vi "e_guidance (SubVI).vi"(9 "Position (i+1)":T1, 10 "Time":T2, 11 "Data":dbl[][](array[numeric])) -> (3 "e(i+1)":dbl[](array[numeric]))   [LabVIEW 2017]
uses:
  <vilib>/Analysis/_algsub.llb/Vector Norm Type.ctl
  <vilib>/Analysis/_algsub.llb/Real Vector Norm.vi
  <vilib>/Analysis/baseanly.llb/Mean (DBL).vi
  <vilib>/Analysis/baseanly.llb/Real Dot Product.vi
  <vilib>/Analysis/Matrix/Numeric/Conversions/Array To Matrix - RA2.vi
  <vilib>/Analysis/Matrix/Numeric/Conversions/Matrix To Array - RM.vi
  <vilib>/Analysis/NI_AALPro.lvlib
  <vilib>/Analysis/NI_AALBase.lvlib
  <vilib>/Analysis/Matrix/NI_Matrix.lvlib
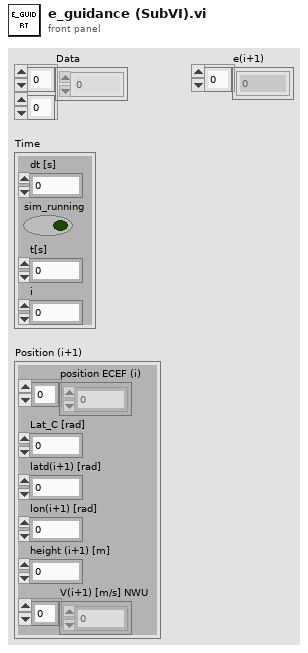
[diagram p1: front panel]
types:
  T1 = cluster{"position ECEF (i)":dbl[], "Lat_C [rad]":dbl, "latd(i+1) [rad]":dbl, "lon(i+1) [rad]":dbl, "height (i+1) [m]":dbl, "V(i+1) [m/s] NWU":dbl[]}
  T2 = cluster{"dt [s]":dbl, "sim_running":bool, "t[s]":dbl, "i":i32}
  T3 = typedef "NI_AALPro.lvlib/Vector Norm Type.ctl" = u16
  T4 = typedef "NI_Matrix.lvlib/RealMatrix.ctl" = dbl[][]
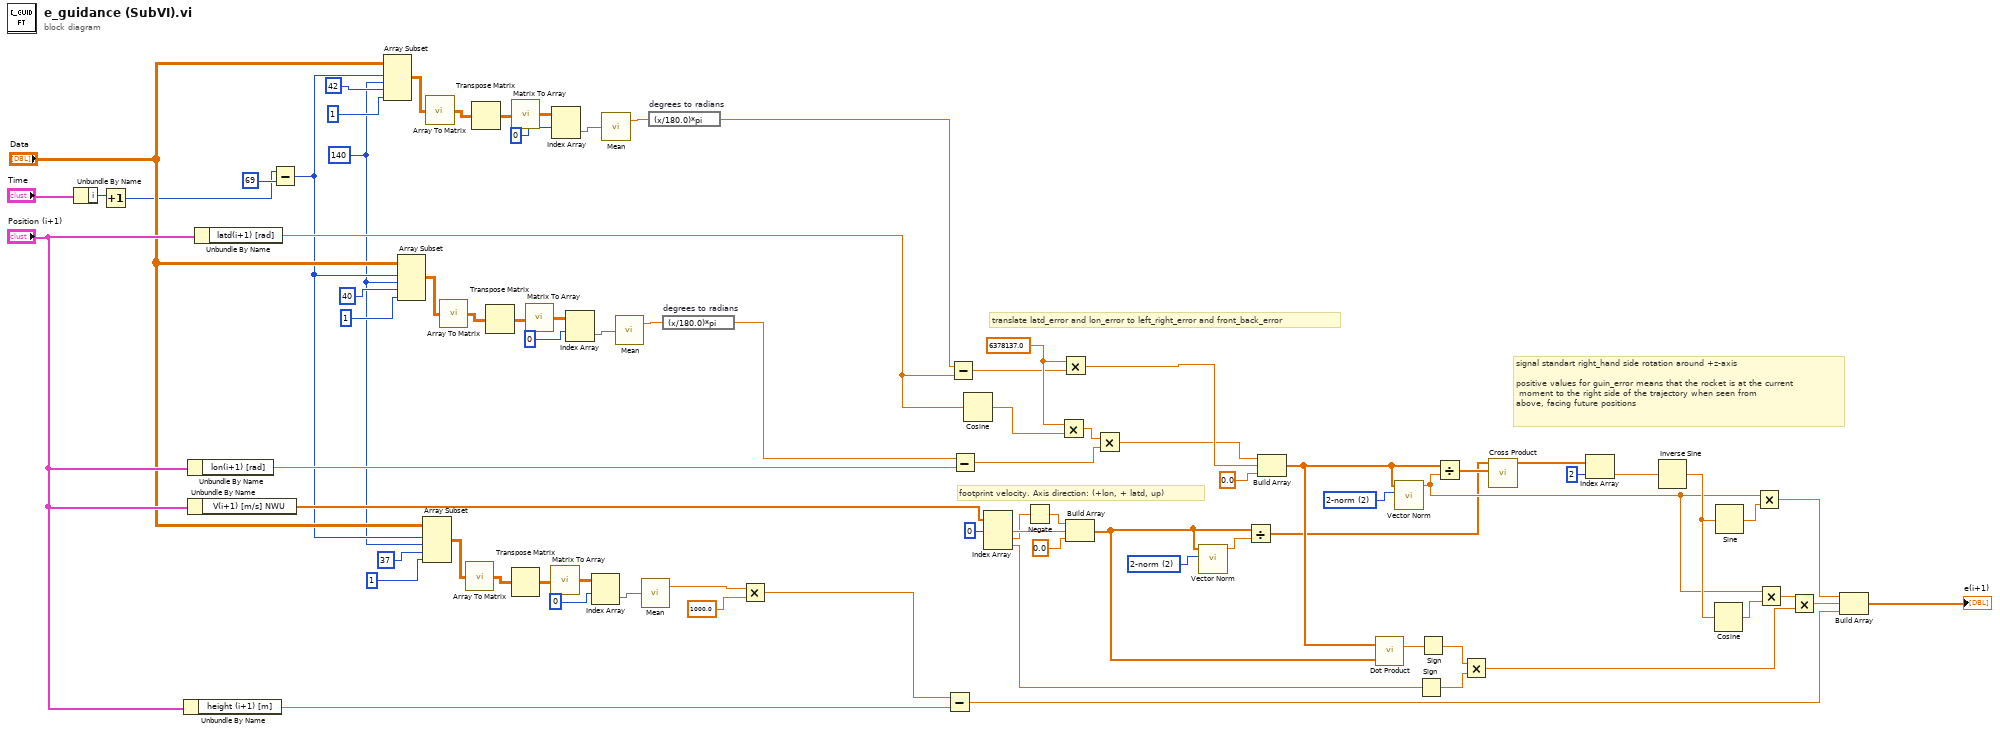
[diagram p0: block diagram]
diagram:
  w6 = 140 ("length")
  w56 = T3 2 items=["1-norm"=1, "2-norm"=2, "Inf-norm"=3, "-Inf-norm"=4, "User Defined"=5] ("norm type")
  w54 = T3 2 items=["1-norm"=1, "2-norm"=2, "Inf-norm"=3, "-Inf-norm"=4, "User Defined"=5] ("norm type")
  w41 = 6378137.0 ("x")
  # "signal standart right_hand side rotation around +z-axis\n\npositive values for guin_error means that the rocket is at the current\n moment to the right side of the trajectory when seen from \nabove, facing future positions"
  # "footprint velocity. Axis direction: (+lon, + latd, up)"
  # "translate latd_error and lon_error to left_right_error and front_back_error"
  n1 = Unbundle By Name("Time") -> ("i"=w74:i32)
  n2 = Increment(x=w74) -> (x+1=w7:i32)
  n3 = Unbundle By Name("Position (i+1)") -> ("height (i+1) [m]"=w75:dbl)
  n4 = Unbundle By Name("Position (i+1)") -> ("lon(i+1) [rad]"=w38:dbl)
  n5 = Unbundle By Name("Position (i+1)") -> ("V(i+1) [m/s] NWU"=w48:dbl[])
  n6 = Unbundle By Name("Position (i+1)") -> ("latd(i+1) [rad]"=w40:dbl)
  n7 = Subtract(x=w7, y=69) -> (x-y=w8:i32)
  n8 = Array Subset(array="Data", index (row)=w8, length (row)=w6, index (col)=42 ("index"), length (col)=1 ("length")) -> (w28:dbl[][])
  n9 = Array Subset(array="Data", index (row)=w8, length (row)=w6, index (col)=40 ("index"), length (col)=1 ("length")) -> (w24:dbl[][])
  n10 = Array Subset(array="Data", index (row)=w8, length (row)=w6, index (col)=37 ("index"), length (col)=1 ("length")) -> (w11:dbl[][])
  n11 = call-poly <vilib>:"Array To Matrix.vi"("Real 2D Array"=w28) -> ("Real Matrix"=w32:T4)
  n12 = call-poly <vilib>:"Array To Matrix.vi"("Real 2D Array"=w24) -> ("Real Matrix"=w21:T4)
  n13 = call-poly <vilib>:"Array To Matrix.vi"("Real 2D Array"=w11) -> ("Real Matrix"=w14:T4)
  n14 = Transpose Matrix(1:w32) -> (0:w31:T4)
  n15 = Transpose Matrix(1:w21) -> (0:w22:T4)
  n16 = call-poly <vilib>:"Matrix To Array.vi"("Real Matrix"=w31) -> ("Real 2D Array"=w30:dbl[][])
  n17 = Transpose Matrix(1:w14) -> (0:w13:T4)
  n18 = call-poly <vilib>:"Matrix To Array.vi"("Real Matrix"=w22) -> ("Real 2D Array"=w23:dbl[][])
  n19 = call-poly <vilib>:"Matrix To Array.vi"("Real Matrix"=w13) -> ("Real 2D Array"=w12:dbl[][])
  n20 = Index Array(array=w30, index (row)=0) -> (element=w27:dbl[])  [unwired: 1 in]
  n21 = Index Array(array=w23, index (row)=0) -> (element=w25:dbl[])  [unwired: 1 in]
  n22 = Index Array(array=w12, index (row)=0) -> (element=w10:dbl[])  [unwired: 1 in]
  n23 = call-poly <vilib>:"Mean.vi"("X"=w27) -> ("mean"=w5:dbl)  [unwired: 1 out]
  n24 = call-poly <vilib>:"Mean.vi"("X"=w25) -> ("mean"=w4:dbl)  [unwired: 1 out]
  n25 = call-poly <vilib>:"Mean.vi"("X"=w10) -> ("mean"=w2:dbl)  [unwired: 1 out]
  n26 = expression code="(x/180.0)*pi" "degrees to radians"(w5) -> (w26:dbl)
  n27 = expression code="(x/180.0)*pi" "degrees to radians"(w4) -> (w36:dbl)
  n28 = Multiply(x=w2, y=1000.0) -> (x*y=w1:dbl)
  n29 = Subtract(x=w1, y=w75) -> (x-y=w79:dbl)
  n30 = Subtract(x=w26, y=w40) -> (x-y=w39:dbl)
  n31 = Subtract(x=w36, y=w38) -> (x-y=w44:dbl)
  n32 = Cosine(x=w40) -> (cos(x)=w42:dbl)
  n33 = Index Array(array=w48, index #1=0 ("index")) -> (element #1=w52:dbl, element #2=w51:dbl, element #3=w69:dbl)  [unwired: 2 in]
  n34 = Negate(x=w51) -> (-x=w50:dbl)
  n35 = Multiply(x=w41, y=w42) -> (x*y=w43:dbl)
  n36 = Multiply(x=w41, y=w39) -> (x*y=w46:dbl)
  n37 = Build Array(w50, w52, 0.0 ("element")) -> (w67:dbl[])
  n38 = Multiply(x=w43, y=w44) -> (x*y=w45:dbl)
  n39 = call-poly <vilib>:"Vector Norm.vi"("norm type"=w54, "Input Vector"=w67) -> ("norm"=w55:dbl)  [unwired: 8 in, 1 out]
  n40 = Divide(x=w67, y=w55) -> (x/y=w57:dbl[])
  n41 = Build Array(w45, w46, 0.0 ("element")) -> (w66:dbl[])
  n42 = call-poly <vilib>:"Dot Product.vi"("Y Vector"=w67, "X Vector"=w66) -> ("X * Y"=w68:dbl)  [unwired: 1 out]
  n43 = call-poly <vilib>:"Vector Norm.vi"("norm type"=w56, "Input Vector"=w66) -> ("norm"=w63:dbl)  [unwired: 8 in, 1 out]
  n44 = Sign(1:w69) -> (0:w71:dbl)
  n45 = Sign(1:w68) -> (0:w70:dbl)
  n46 = Divide(x=w66, y=w63) -> (x/y=w58:dbl[])
  n47 = Multiply(x=w70, y=w71) -> (x*y=w73:dbl)
  n48 = call <vilib>:"Cross Product.vi"("B Vector"=w58, "A Vector"=w57) -> ("Cross Product"=w61:dbl[])  [unwired: 8 in, 1 out]
  n49 = Index Array(array=w61, index=2) -> (element=w62:dbl)
  n50 = Inverse Sine(1:w62) -> (0:w65:dbl)
  n51 = Cosine(x=w65) -> (cos(x)=w64:dbl)
  n52 = Sine(x=w65) -> (sin(x)=w59:dbl)
  n53 = Multiply(x=w63, y=w59) -> (x*y=w77:dbl)
  n54 = Multiply(x=w63, y=w64) -> (x*y=w72:dbl)
  n55 = Multiply(x=w72, y=w73) -> (x*y=w78:dbl)
  n56 = Build Array(w77, w78, w79) -> (→"e(i+1)":dbl[])
